vi "Undo States.vi"(8 "error in":errorcluster, 10 "Expected Undo States":string[](array[string]), 11 "Test Case In":refnum<class "Undo Redo Core.lvclass">) -> (0 "error out":errorcluster, 1 "Final Have Changes":bool, 2 "Actual Undo States":string[](array[string]), 3 "Test Case Out":refnum<class "Undo Redo Core.lvclass">)   [LabVIEW 2021, in "Undo Redo Core.lvclass"]
uses:
  Undo Redo Core.lvclass
  C:/Program Files/National Instruments/LabVIEW 2024/vi.lib/Astemes/LUnit/Test Case.lvclass
  <resource>/plugins/NIIconEditor/Controls/Undo Redo Action.ctl
  <vilib>/Astemes/LUnit/Test Case.lvclass/Test Case.ctl
  c447cda1-e09e-4100-8da7-89a8f417bcef.vi
  <vilib>/Astemes/LUnit/Append Pass Result.vi
  <vilib>/Astemes/LUnit/Append Fail Result.vi
  c447cda1-e09e-4100-8da7-89a8f417bcef.vi/9c5d11cd-9439-4240-a1ee-d9baace9c924.vi
  <vilib>/Astemes/LUnit/Run In UI.vi
  <vilib>/Utility/error.llb/Clear Errors.vi
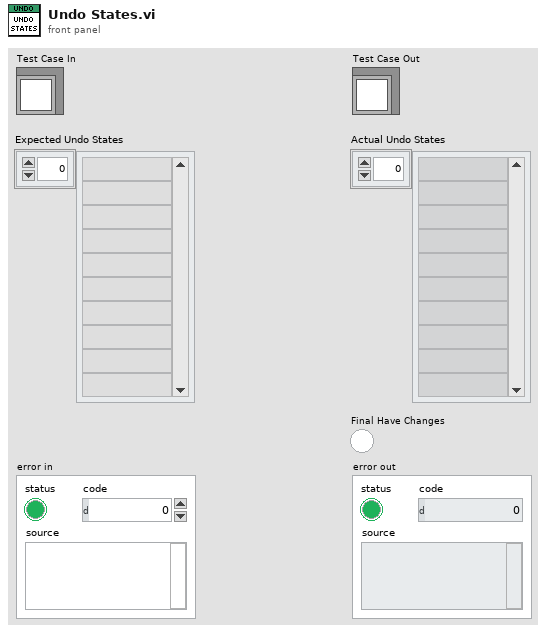
[diagram p1: front panel]
types:
  T1 = typedef "Undo Redo Action.ctl" = enum16{"Init", "Add", "Undo", "Redo", "Current State"}
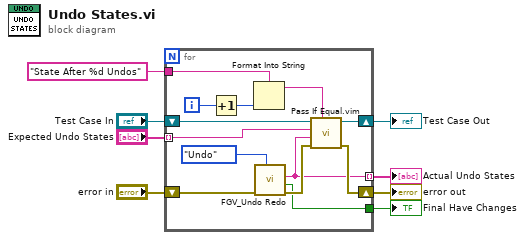
[diagram p0: block diagram]
diagram:
  n1 = for {
    tunnel: [w14] -> w3 mode=indexing
    shift-right: [w15] -> w5
    shift-left: "Test Case In" -> [w16]
    tunnel: "Expected Undo States" -> [w17] mode=indexing
    shift-right: [w21] -> w7
    shift-left: "error in" -> [w19]
    tunnel: "State After %d Undos" ("Description") -> [w11]
    tunnel: [w9] -> w1
    i -> [w13]
    n2 = Increment(x=w13) -> (x+1=w10:i32)
    n3 = Format Into String(format string=w11, w10) -> (resulting string=w12:string)  [unwired: 2 in, 1 out]
    n4 = call <resource>:"FGV_Undo Redo.vi"("Action"=Undo_Redo_Action."Undo", "error in"=w19) -> ("error out"=w20:errorcluster, "Have Changes"=w9:bool, "State Out"=w14:string)  [unwired: 7 in]
    n5 = call "Pass If Equal.vim"("Description"=w12, "error in (no error)"=w20, "Actual"=w14, "Expected"=w17, "LUnit Test Case In"=w16) -> ("error out"=w21:errorcluster, "LUnit Test Case Out"=w15:refnum<class "Undo Redo Core.lvclass">)  [unwired: 5 in]
  }
  "Test Case Out" <- w5
  "error out" <- w7
  "Actual Undo States" <- w3
  "Final Have Changes" <- w1
